vi "追溯Global.vi"() -> ()   [LabVIEW 2018]
panel:
  out "DEVICE_ID":i64
  out "USER_ID":i64
  out "PRODUCT_ID":i64
  out "CODE_ID":i64
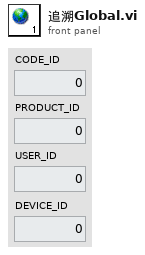
[diagram p1: front panel]
diagram:
